vi "test read api.vi"() -> ()   [LabVIEW 2019]
uses:
  <vilib>/httpClient/POSTBuffer.vi
  <vilib>/httpClient/LabVIEWHTTPClient.lvlib
panel:
  out "JSON string":string
  out "Table Control":string[][](table)
  out "value":T1
  out "body":string
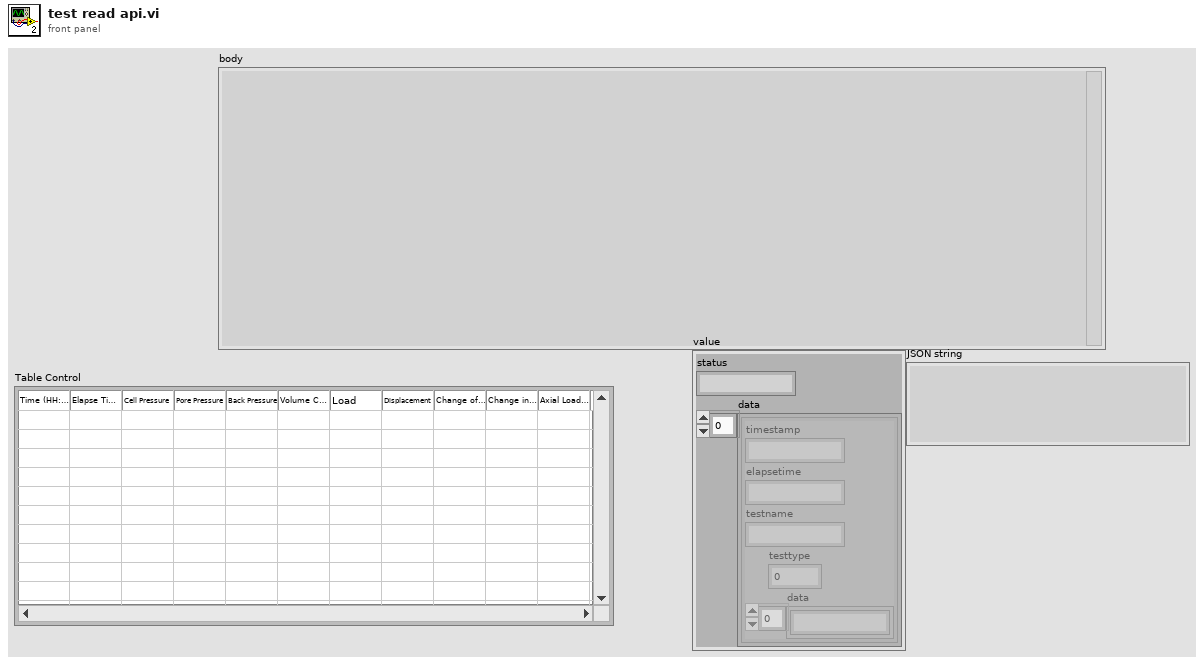
[diagram p1: front panel]
types:
  T1 = cluster{"status":string, "data":cluster{"timestamp":string, "elapsetime":string, "testname":string, "testtype":u16, "data":string[]}[]}
  T2 = cluster{"testtype":u16, "testname":string, "fileid":string}
  T3 = typedef "LabVIEWHTTPClient.lvlib/ClientHandle.ctl" = refnum<k1>
  T4 = cluster{"timestamp":string, "elapsetime":string, "testname":string, "testtype":u16, "data":string[]}[]
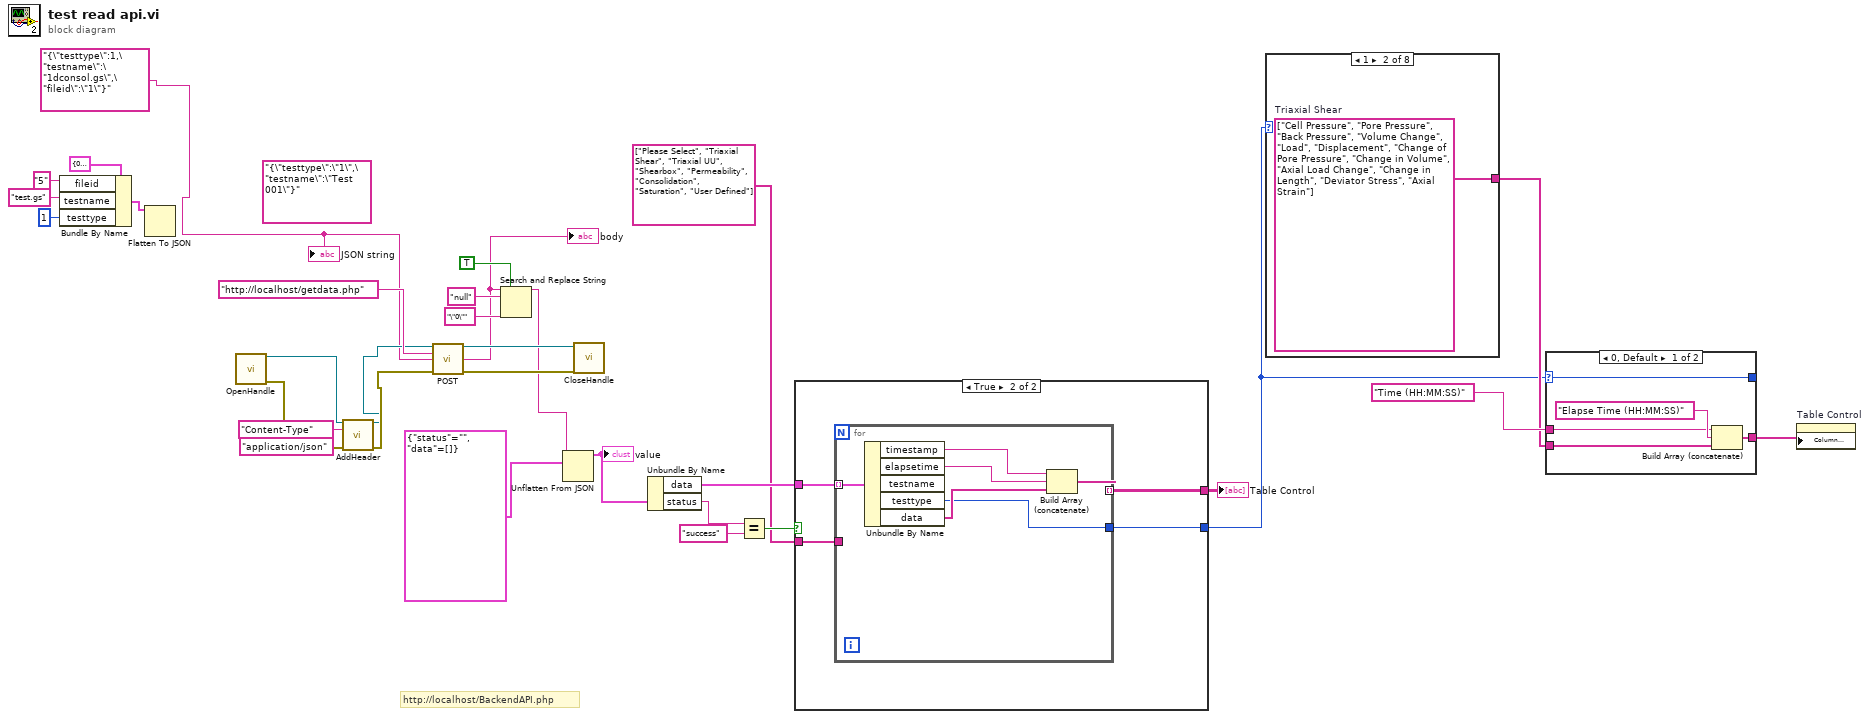
[diagram p0: block diagram]
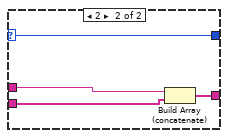
[diagram p2: hidden frame]
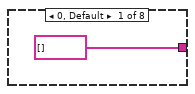
[diagram p3: hidden frame]
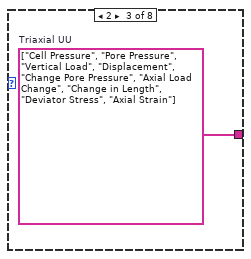
[diagram p4: hidden frame]
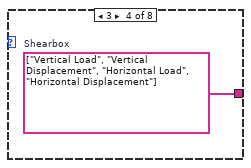
[diagram p5: hidden frame]
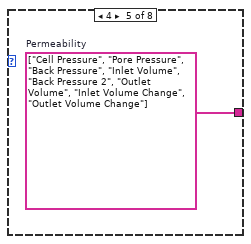
[diagram p6: hidden frame]
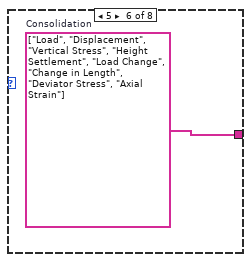
[diagram p7: hidden frame]
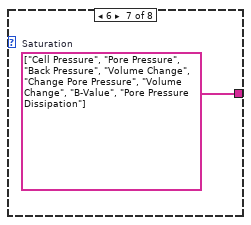
[diagram p8: hidden frame]
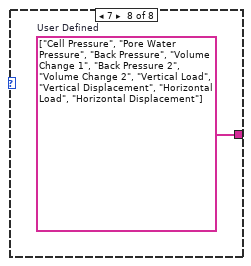
[diagram p9: hidden frame]
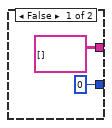
[diagram p10: hidden frame]
diagram:
  w6 = "{\"testtype\":1,\"testname\":\"1dconsol.gs\",\"fileid\":\"1\"}" ("buffer")
  (unwired) "{\"testtype\":\"1\",\"testname\":\"Test 001\"}" ("buffer")
  # "http://localhost/BackendAPI.php"
  n1 = Bundle By Name(cluster=T2 {"testtype"=0, "testname"="", "fileid"=""}, "fileid"="5", "testname"="test.gs", "testtype"=u16 1) -> (w15:T2)
  n2 = Flatten To JSON(anything=w15) -> ()  [unwired: 2 in, 2 out]
  n3 = call <vilib>:"OpenHandle.vi"() -> ("client handle out"=w27:T3, "error out"=w29:errorcluster)  [unwired: 14 in]
  n4 = call <vilib>:"AddHeader.vi"("client handle"=w27, "header"="Content-Type", "value"="application/json", "error in (no error)"=w29) -> ("client handle out"=w26:T3, "error out"=w28:errorcluster)  [unwired: 10 in]
  n5 = call-poly <vilib>:"POST.vi"("client handle"=w26, "url"="http://localhost/getdata.php", "buffer"=w6, "error in (no error)"=w28) -> ("client handle out"=w31:T3, "body"=w2:string, "error out"=w32:errorcluster)  [unwired: 8 in, 1 out]
  "body" <- w2
  n6 = Search and Replace String(replace all?=TRUE ("replace all? (F)"), input string=w2, search string="null", replace string="\"0\"" ("replace string (\"\")")) -> (result string=w1:string)  [unwired: 4 in, 3 out]
  n7 = Unflatten From JSON(JSON string=w1, type and defaults=T1 {"status"="", "data"=[]}) -> (value=w22:T1)  [unwired: 5 in, 1 out]
  "value" <- w22
  n8 = call <vilib>:"CloseHandle.vi"("client handle"=w31, "error in (no error)"=w32) -> ()  [unwired: 13 in, 1 out]
  n9 = Unbundle By Name(w22) -> ("data"=w18:T4, "status"=w21:string)
  n10 = Equal?(x=w21, y="success") -> (x = y?=w19:bool)
  n11 = case shown="True" w19 {
    tunnel: w18 -> [_ w38]
    tunnel: [string[][] [] w37] -> w17
    tunnel: string[] ["Please Select", "Triaxial Shear", "Triaxial UU", "Shearbox", "Permeability", "Consolidation", "Saturation", "User Defined"] ("Strings []") -> [_ w36]
    tunnel: [u16 0 ("testtype") w35] -> w8
    frame False {
    }
    frame True {
      n12 = for {
        tunnel: w38 -> [w44] mode=indexing
        tunnel: [w40] -> w37 mode=indexing
        tunnel: w36 -> [_]
        tunnel: [w39] -> w35
        n13 = Unbundle By Name(w44) -> ("timestamp"=w43:string, "elapsetime"=w42:string, "testtype"=w39:u16, "data"=w41:string[])  [unwired: 1 out]
        n14 = Build Array (concatenate)(w43, w42, w41) -> (w40:string[])
      }
    }
  }
  "Table Control" <- w17
  n15 = case shown="1" w8 {
    tunnel: [string[] [] w46 w47 w48 w49 w50 w51 w52] -> w9
    frame 0, Default {
    }
    frame 1 {
      w46 = string[] ["Cell Pressure", "Pore Pressure", "Back Pressure", "Volume Change", "Load", "Displacement", "Change of Pore Pressure", "Change in Volume", "Axial Load Change", "Change in Length", "Deviator Stress", "Axial Strain"]  # Triaxial Shear
    }
    frame 2 {
      w47 = string[] ["Cell Pressure", "Pore Pressure", "Vertical Load", "Displacement", "Change Pore Pressure", "Axial Load Change", "Change in Length", "Deviator Stress", "Axial Strain"]  # Triaxial UU
    }
    frame 3 {
      w48 = string[] ["Vertical Load", "Vertical Displacement", "Horizontal Load", "Horizontal Displacement"]  # Shearbox
    }
    frame 4 {
      w49 = string[] ["Cell Pressure", "Pore Pressure", "Back Pressure", "Inlet Volume", "Back Pressure 2", "Outlet Volume", "Inlet Volume Change", "Outlet Volume Change"]  # Permeability
    }
    frame 5 {
      w50 = string[] ["Load", "Displacement", "Vertical Stress", "Height Settlement", "Load Change", "Change in Length", "Deviator Stress", "Axial Strain"]  # Consolidation
    }
    frame 6 {
      w51 = string[] ["Cell Pressure", "Pore Pressure", "Back Pressure", "Volume Change", "Change Pore Pressure", "Volume Change", "B-Value", "Pore Pressure Dissipation"]  # Saturation
    }
    frame 7 {
      w52 = string[] ["Cell Pressure", "Pore Water Pressure", "Back Pressure", "Volume Change 1", "Back Pressure 2", "Volume Change 2", "Vertical Load", "Vertical Displacement", "Horizontal Load", "Horizontal Displacement"]  # User Defined
    }
  }
  n16 = case shown="0, Default" w8 {
    selector: w8 -> [w53 w58]
    tunnel: "Time (HH:MM:SS)" ("element") -> [w56 w61]
    tunnel: w9 -> [w55 w60]
    tunnel: [w54 w59] -> w7
    tunnel: [w53 w58] -> _
    frame 0, Default {
      n17 = Build Array (concatenate)(w56, "Elapse Time (HH:MM:SS)" ("String"), w55) -> (w54:string[])
    }
    frame 2 {
      n18 = Build Array (concatenate)(w61, w60) -> (w59:string[])
    }
  }
  n19 = property on="Table Control" class="Tbl (strict)"("Column Headers[]"=w7) -> ()  [unwired: 2 in, 2 out]
  "JSON string" <- w6
